vi "S&E to String.vi"(7 "E&S Message in":T1, 11 "error in":errorcluster) -> (4 "date/time string":string, 6 "Location/ID":string, 8 "File Header":string, 10 "Data":string, 14 "Value":string, 15 "error Out":errorcluster)   [LabVIEW 2011]
uses:
  emi Lib/System 01/0 - General/S&E reporting/Private/_emi_ S&E Message.ctl
  emi Lib/System 01/0 - General/S&E reporting/Private/_emi_ S&E Message type.ctl
  Measurments Handling/Action Analog Handler.ctl
panel:
  in  "Digital values":bool[](array[boolean])
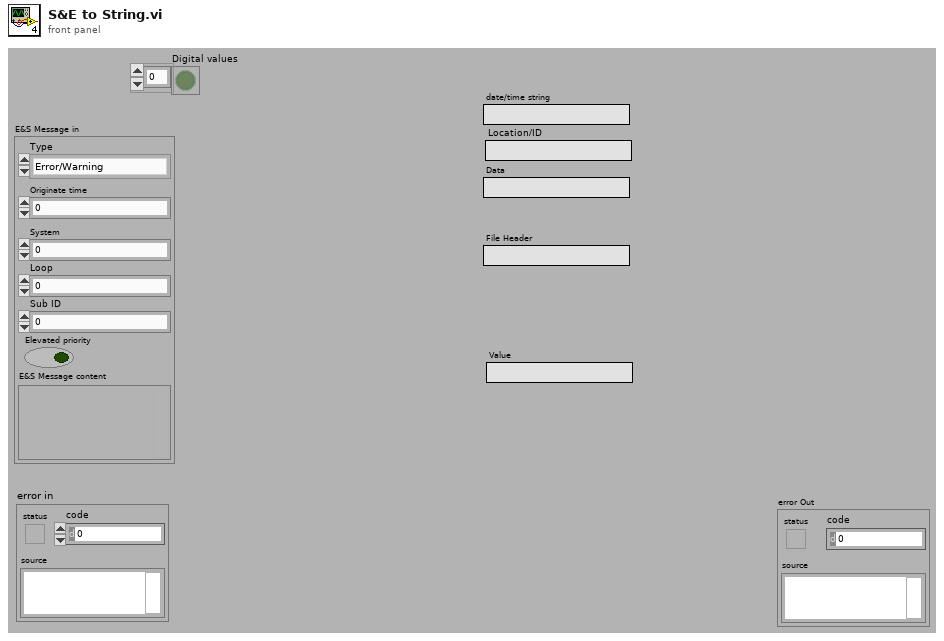
[diagram p1: front panel]
types:
  T1 = typedef "_emi_ S&E Message.ctl" = cluster{"Type":T2, "Originate time":dbl, "System":u8, "Loop":u16, "Sub ID":u16, "Elevated priority":bool, "E&S Message content":variant}
  T2 = typedef "_emi_ S&E Message type.ctl" = enum16{"Error/Warning", "Note", "Debug", "Event", "Alarm Analog", "Alarm Digital", "Annotation"}
  T3 = typedef "Action Analog Handler.ctl" = enum16{"GET value", "GET Single Frequenzy", "GET All Values", "GET Waveform", "Get Numb Var", "SET Value", "START Buffer", "REG Variable", "BUF size(total antal sekund)", "PULS", "Get a Value at time", "Set initial waveform"}
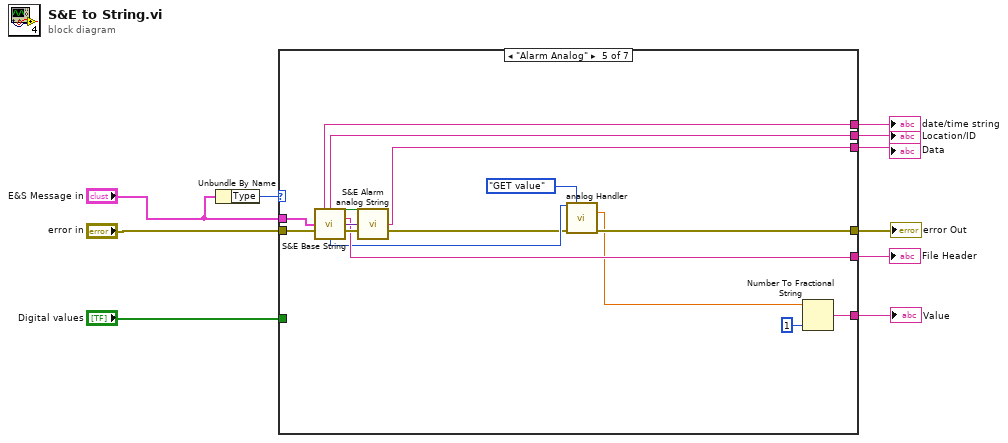
[diagram p0: block diagram]
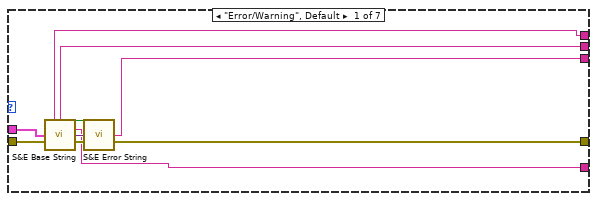
[diagram p2: hidden frame]
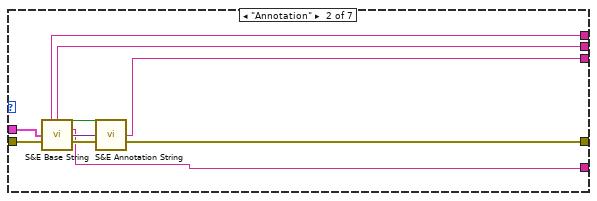
[diagram p3: hidden frame]
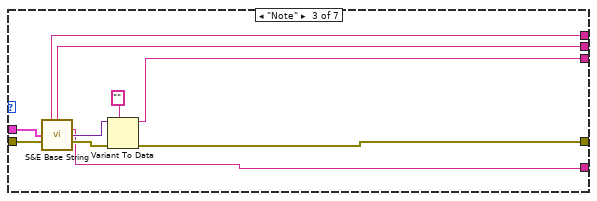
[diagram p4: hidden frame]
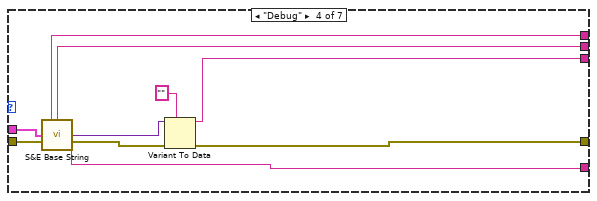
[diagram p5: hidden frame]
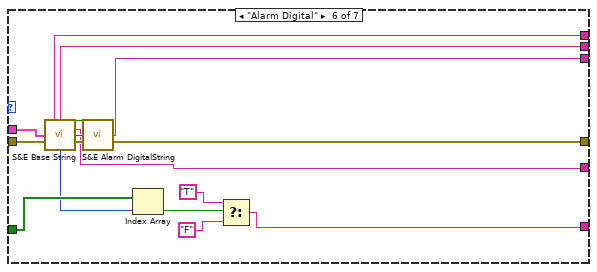
[diagram p6: hidden frame]
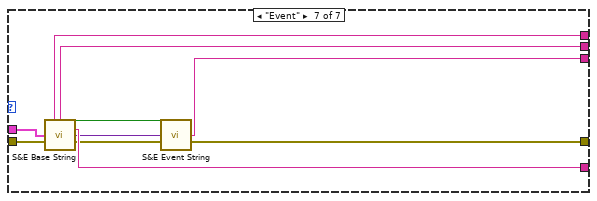
[diagram p7: hidden frame]
diagram:
  n1 = Unbundle By Name("E&S Message in") -> ("Type"=w10:T2)
  n2 = case shown="\"Alarm Analog\"" w10 {
    tunnel: "error in" -> [w16 w29 w39 w49 w65 w81 w91]
    tunnel: [w15 w25 w37 w47 w52 w77 w86] -> w7
    tunnel: "E&S Message in" -> [w20 w30 w40 w50 w66 w82 w92]
    tunnel: [w11 w21 w31 w41 w58 w73 w90] -> w6
    tunnel: [w14 w24 w33 w44 w61 w76 w85] -> w5
    tunnel: [w13 w23 w32 w43 w60 w75 w84] -> w4
    tunnel: [w12 w22 w34 w42 w59 w74 w83] -> w3
    tunnel: [_ _ _ _ w56 w67 _] -> w2
    tunnel: "Digital values" -> [_ _ _ _ _ w72 _]
    frame "Error/Warning", Default {
      n3 = call "S&E Base String.vi"("E&S Message"=w20, "error in (no error)"=w16) -> ("date/time string"=w14:string, "Location/ID"=w13:string, "Elevated priority"=w17:bool, "Measage text file Header string"=w11:string, "Message content"=w19:variant, "error out"=w18:errorcluster)  [unwired: 6 in, 2 out]
      n4 = call "S&E Error String.vi"("Elevated priority"=w17, "Content"=w19, "error in"=w18) -> ("format string"=w12:string, "error out"=w15:errorcluster)  [unwired: 11 in]
    }
    frame "Annotation" {
      n5 = call "S&E Base String.vi"("E&S Message"=w30, "error in (no error)"=w29) -> ("date/time string"=w24:string, "Location/ID"=w23:string, "Elevated priority"=w26:bool, "Measage text file Header string"=w21:string, "Message content"=w27:variant, "error out"=w28:errorcluster)  [unwired: 6 in, 2 out]
      n6 = call "S&E Annotation String.vi"("Elevated priority"=w26, "Content"=w27, "error in"=w28) -> ("format string"=w22:string, "error out"=w25:errorcluster)  [unwired: 11 in]
    }
    frame "Note" {
      n7 = call "S&E Base String.vi"("E&S Message"=w40, "error in (no error)"=w39) -> ("date/time string"=w33:string, "Location/ID"=w32:string, "Measage text file Header string"=w31:string, "Message content"=w35:variant, "error out"=w38:errorcluster)  [unwired: 6 in, 3 out]
      n8 = Variant To Data(error in=w38, type="" ("Measage Header string"), Variant=w35) -> (data=w34:string, error out=w37:errorcluster)
    }
    frame "Debug" {
      n9 = call "S&E Base String.vi"("E&S Message"=w50, "error in (no error)"=w49) -> ("date/time string"=w44:string, "Location/ID"=w43:string, "Measage text file Header string"=w41:string, "Message content"=w45:variant, "error out"=w48:errorcluster)  [unwired: 6 in, 3 out]
      n10 = Variant To Data(error in=w48, type="" ("Measage Header string"), Variant=w45) -> (data=w42:string, error out=w47:errorcluster)
    }
    frame "Alarm Analog" {
      n11 = call "S&E Base String.vi"("E&S Message"=w66, "error in (no error)"=w65) -> ("date/time string"=w61:string, "Location/ID"=w60:string, "Elevated priority"=w62:bool, "Measage text file Header string"=w58:string, "Message content"=w63:variant, "error out"=w64:errorcluster, "Sub ID"=w54:u16)  [unwired: 6 in, 1 out]
      n12 = call "S&E Alarm analog String.vi"("Elevated priority"=w62, "Content"=w63, "error in"=w64) -> ("format string"=w59:string, "error out"=w53:errorcluster)  [unwired: 11 in]
      n13 = call "analog Handler.vi"("Variable Index"=w54, "Action"=Action_Analog_Handler."GET value", "error in (no error)"=w53) -> ("Value out"=w51:dbl, "error out"=w52:errorcluster)  [unwired: 7 in, 4 out]
      n14 = Number To Fractional String(number=w51, precision (6)=i16 1) -> (F-format string=w56:string)  [unwired: 2 in]
    }
    frame "Alarm Digital" {
      n15 = call "S&E Base String.vi"("E&S Message"=w82, "error in (no error)"=w81) -> ("date/time string"=w76:string, "Location/ID"=w75:string, "Elevated priority"=w78:bool, "Measage text file Header string"=w73:string, "Message content"=w79:variant, "error out"=w80:errorcluster, "Sub ID"=w71:u16)  [unwired: 6 in, 1 out]
      n16 = call "S&E Alarm DigitalString.vi"("Elevated priority"=w78, "Content"=w79, "error in"=w80) -> ("format string"=w74:string, "error out"=w77:errorcluster)  [unwired: 11 in]
      n17 = Index Array(array=w72, index=w71) -> (element=w70:bool)
      n18 = Select(t="T", s=w70, f="F") -> (s? t:f=w67:string)
    }
    frame "Event" {
      n19 = call "S&E Base String.vi"("E&S Message"=w92, "error in (no error)"=w91) -> ("date/time string"=w85:string, "Location/ID"=w84:string, "Elevated priority"=w87:bool, "Measage text file Header string"=w90:string, "Message content"=w88:variant, "error out"=w89:errorcluster)  [unwired: 6 in, 2 out]
      n20 = call "S&E Event String.vi"("Elevated priority"=w87, "Content"=w88, "error in"=w89) -> ("format string"=w83:string, "error out"=w86:errorcluster)  [unwired: 11 in]
    }
  }
  "error Out" <- w7
  "File Header" <- w6
  "date/time string" <- w5
  "Location/ID" <- w4
  "Data" <- w3
  "Value" <- w2
